vi "Send Swap Controllers.vi"(7 "消息优先级（标准）":T1=enum."Normal", 8 "error in (no error)":cluster{"状态":bool, "代码":i32, "源":string} caption="错误输入（无错误）", 10 "冷却器控制器":refnum<class "Cooler Controller.lvclass">, 11 "消息待入队列":refnum<class "Message Enqueuer.lvclass">) -> (0 "error out":cluster{"状态":bool, "代码":i32, "源":string} caption="错误输出")   [LabVIEW 2013, in "Air Cooler Application.lvlib" / "Swap Controllers Msg.lvclass"]
doc: "本VI将消息发送至操作者。输入用于指定待启动的控制器。"
uses:
  Swap Controllers Msg.lvclass
  <vilib>/ActorFramework/Message Enqueuer/Message Enqueuer.lvclass
  <vilib>/ActorFramework/Message Enqueuer/Message Priority.ctl
  Cooler Controller/Cooler Controller/Cooler Controller.lvclass
  Swap Controllers Msg.lvclass/Swap Controllers Msg.ctl
  <vilib>/ActorFramework/Message Enqueuer/Message Enqueuer.lvclass/Message Enqueuer.ctl
  <vilib>/ActorFramework/Message Priority Queue/Priority Enqueue.vi
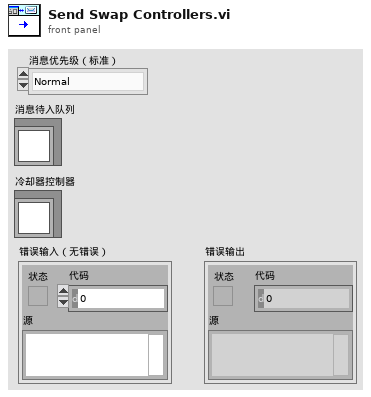
[diagram p1: front panel]
types:
  T1 = typedef "Actor Framework.lvlib/Message Enqueuer.lvclass/Message Priority.ctl" = enum16{"Low", "Normal", "High"}
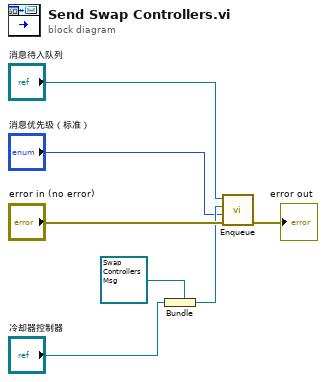
[diagram p0: block diagram]
diagram:
  n1 = Bundle(cluster=refnum<class "Swap Controllers Msg.lvclass"> refnum ("Object"), "冷却器控制器") -> (w3:refnum<class "Swap Controllers Msg.lvclass">)
  n2 = call <vilib>:"Enqueue.vi"("error in (no error)"="error in (no error)", "Message Priority (Normal)"="消息优先级（标准）", "Message"=w3, "Message Enqueuer in"="消息待入队列") -> ("error out"=→"error out":errorcluster)  [unwired: 6 in, 1 out]
